vi "Configure Period.vi"(8 "error in (no error)":errorcluster, 10 "period, s":dbl format="%#_6p", 11 "TroSpec in":refnum<class "PL ISTEQ TroSpec.lvclass">) -> (0 "error out":errorcluster, 3 "TroSpec out":refnum<class "PL ISTEQ TroSpec.lvclass">)   [LabVIEW 2015, in "PL ISTEQ TroSpec.lvclass"]
doc: "Configures CCD acquisition period."
uses:
  PL ISTEQ TroSpec.lvclass
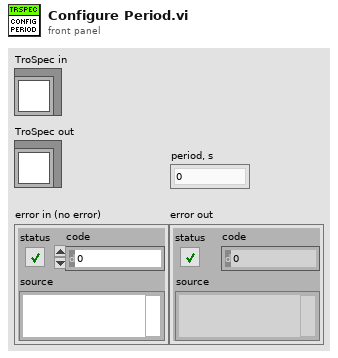
[diagram p1: front panel]
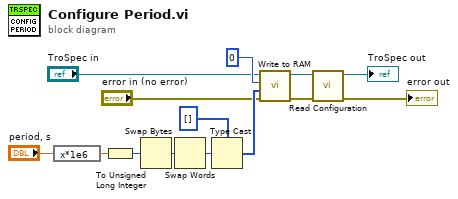
[diagram p0: block diagram]
diagram:
  n1 = expression code="x*1e6"("period, s") -> (w13:dbl)
  n2 = To Unsigned Long Integer(number=w13) -> (unsigned 32bit integer=w12:u32)
  n3 = Swap Bytes(anything=w12) -> (byte swapped=w9:u32)
  n4 = Swap Words(1:w9) -> (0:w8:u32)
  n5 = Type Cast(type=u8[] [] ("data"), x=w8) -> (*(type *) &x=w11:u8[])
  n6 = call "Write to RAM.vi"("error in (no error)"="error in (no error)", "data"=w11, "address"=u16 0, "TroSpec in"="TroSpec in") -> ("error out"=w3:errorcluster, "TroSpec out"=w4:refnum<class "PL ISTEQ TroSpec.lvclass">)  [unwired: 6 in]
  n7 = call "Read Configuration.vi"("error in (no error)"=w3, "TroSpec in"=w4) -> ("error out"=→"error out":errorcluster, "TroSpec out"=→"TroSpec out":refnum<class "PL ISTEQ TroSpec.lvclass">)  [unwired: 7 in, 1 out]
